vi "HEI_Data.vi"(0 "params":dbl[](array[numeric])) -> (7 "Waveform Chart 8":dynamicdata(graph), 8 "RPM":dbl, 9 "Dynamic Data":dynamicdata(waveform), 10 "RPM 2":dbl format="RPM:          %#_g", 11 "RPM 6":dbl format="RPM:          %#_g", 12 "Torque 4":dbl format="Torque:      %#_g", 13 "Torque 2":dbl format="Torque:      %#_g", 14 "Waveform Chart 4":dynamicdata(graph), 15 "Torque 3":dbl, 16 "Torque":dbl, 17 "RPM 4":dbl, 18 "Waveform Chart 6":dynamicdata(graph))   [LabVIEW 2017]
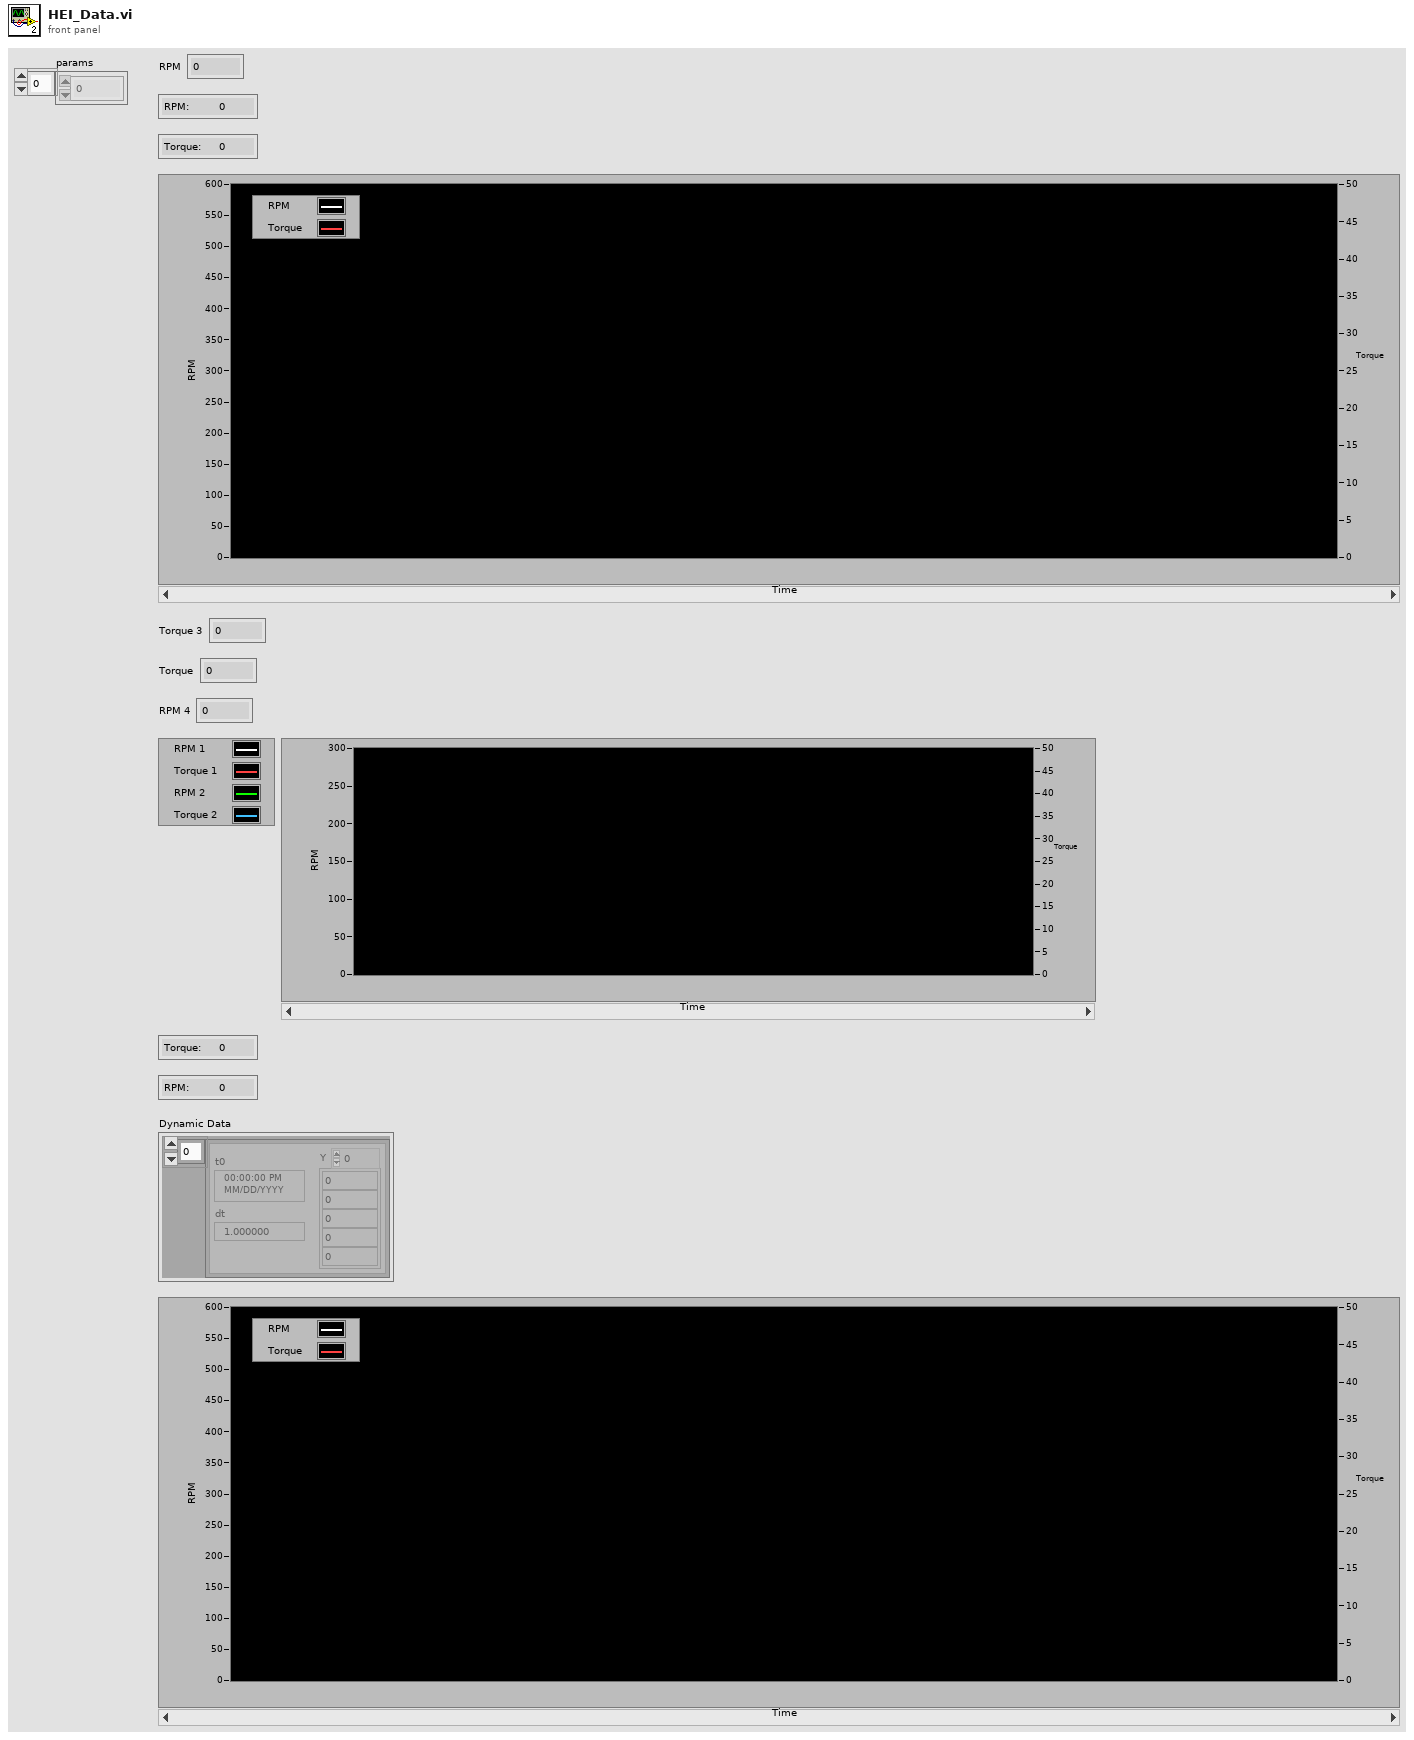
[diagram p1: front panel]
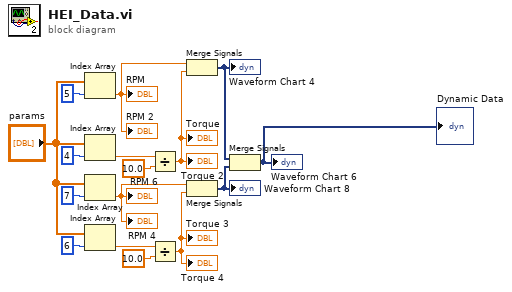
[diagram p0: block diagram]
diagram:
  n1 = Index Array(array="params", index=5) -> (element=w6:dbl)
  "RPM" <- w6
  "RPM 2" <- w6
  n2 = Index Array(array="params", index=4) -> (element=w4:dbl)
  n3 = Index Array(array="params", index=7) -> (element=w15:dbl)
  "RPM 4" <- w15
  "RPM 6" <- w15
  n4 = Index Array(array="params", index=6) -> (element=w10:dbl)
  n5 = Divide(x=w4, y=10.0) -> (x/y=w7:dbl)
  "Torque" <- w7
  "Torque 2" <- w7
  n6 = Divide(x=w10, y=10.0) -> (x/y=w16:dbl)
  "Torque 3" <- w16
  "Torque 4" <- w16
  n7 = Merge Signals(w6, w7) -> (w13:dynamicdata)
  "Waveform Chart 4" <- w13
  n8 = Merge Signals(w15, w16) -> (w14:dynamicdata)
  "Waveform Chart 8" <- w14
  n9 = Merge Signals(w13, w14) -> (→"Waveform Chart 6" →"Dynamic Data":dynamicdata)
